vi "TestStaleInsertIntoPanel_Reject.vi"(8 "error in (no error)":errorcluster, 11 "TestCase in":refnum<class "TestProtectedSubpanel.lvclass">) -> (0 "error out":errorcluster, 3 "TestCase out":refnum<class "TestProtectedSubpanel.lvclass">)   [LabVIEW 2015, in "ProtectedSubpanel.lvlib" / "TestProtectedSubpanel.lvclass"]
uses:
  TestProtectedSubpanel.lvclass
  ProtectedSubpanel.lvclass
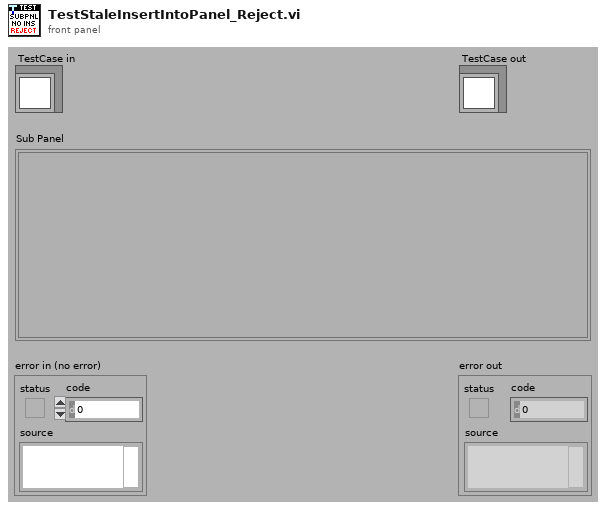
[diagram p1: front panel]
types:
  T1 = typedef "ProtectedSubpanel.lvlib/ProtectedSubpanel.lvclass/Protected Subpanel Reference.ctl" = refnum<data-value>
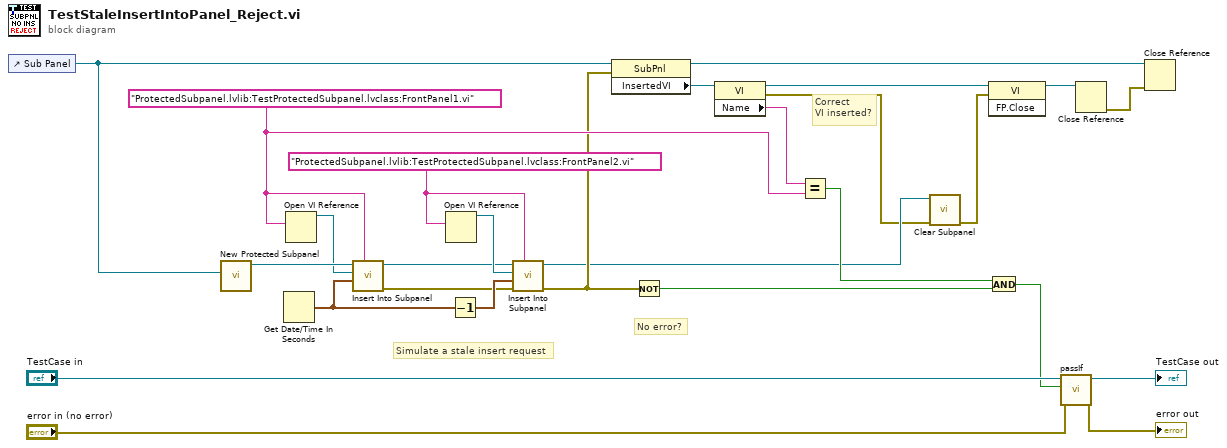
[diagram p0: block diagram]
diagram:
  w16 = "ProtectedSubpanel.lvlib:TestProtectedSubpanel.lvclass:FrontPanel2.vi"
  w14 = "ProtectedSubpanel.lvlib:TestProtectedSubpanel.lvclass:FrontPanel1.vi"
  # "Simulate a stale insert request"
  # "No error?"
  # "Correct\nVI inserted?"
  n1 = control-ref of="Sub Panel"() -> (w10:refnum<vi>)
  n2 = call "New Protected Subpanel.vi"("SubPnl Refnum"=w10) -> ("Protected Subpanel"=w23:T1)  [unwired: 9 in, 1 out]
  n3 = Get Date/Time In Seconds() -> (seconds since 1Jan1904=w12:timestamp)
  n4 = Open VI Reference(vi path=w14) -> (vi reference=w22:refnum<vi>)  [unwired: 5 in, 1 out]
  n5 = call "Insert Into Subpanel.vi"("Viewable Name"=w14, "Insertion Request Time"=w12, "VI Refnum"=w22, "Protected Subpanel"=w23) -> ("error out"=w9:errorcluster, "Protected Subpanel"=w13:T1)  [unwired: 6 in]
  n6 = Open VI Reference(vi path=w16) -> (vi reference=w15:refnum<vi>)  [unwired: 5 in, 1 out]
  n7 = Decrement(x=w12) -> (x-1=w11:timestamp)
  n8 = call "Insert Into Subpanel.vi"("Viewable Name"=w16, "error in (no error)"=w9, "Insertion Request Time"=w11, "VI Refnum"=w15, "Protected Subpanel"=w13) -> ("error out"=w8:errorcluster, "Protected Subpanel"=w5:T1)  [unwired: 5 in]
  n9 = property class="SubPnl"(reference=w10, error in=w8) -> (reference out=w7:refnum<vi>, "InsertedVI"=w20:refnum<vi>)  [unwired: 1 out]
  n10 = Not(x=w8) -> (.not. x?=w21:bool)
  n11 = property class="VI"(reference=w20) -> (reference out=w6:refnum<vi>, error out=w4:errorcluster, "Name"=w18:string)  [unwired: 1 in]
  n12 = Equal?(x=w18, y=w14) -> (x = y?=w17:bool)
  n13 = call "Clear Subpanel.vi"("error in (no error)"=w4, "Protected Subpanel"=w5) -> ("error out"=w1:errorcluster)  [unwired: 8 in, 1 out]
  n14 = invoke class="VI" method="FP.Close"(reference=w6, error in=w1) -> (reference out=w2:refnum<vi>)  [unwired: 1 in, 2 out]
  n15 = And(x=w17, y=w21) -> (x .and. y?=w19:bool)
  n16 = call-dynamic "passIf.vi"("error in (no error)"="error in (no error)", "pass"=w19, "TestCase in"="TestCase in") -> ("error out"=→"error out":errorcluster, "TestCase out"=→"TestCase out":refnum<class "TestProtectedSubpanel.lvclass">)  [unwired: 7 in]
  n17 = Close Reference(reference=w2) -> (error out=w3:errorcluster)  [unwired: 1 in]
  n18 = Close Reference(reference=w7, error in (no error)=w3) -> ()  [unwired: 1 out]
